vi "Controls on Tab.vi"(8 "error in (no error)":errorcluster, 11 "VI Refnum in":refnum<vi>) -> (0 "error out":errorcluster, 2 "ControlOnPages":refnum<vi>[][](array[refnum]), 3 "VI Refnum out":refnum<vi>)   [LabVIEW 2017, in "Toolbox.lvlib"]
uses:
  Toolbox.lvlib
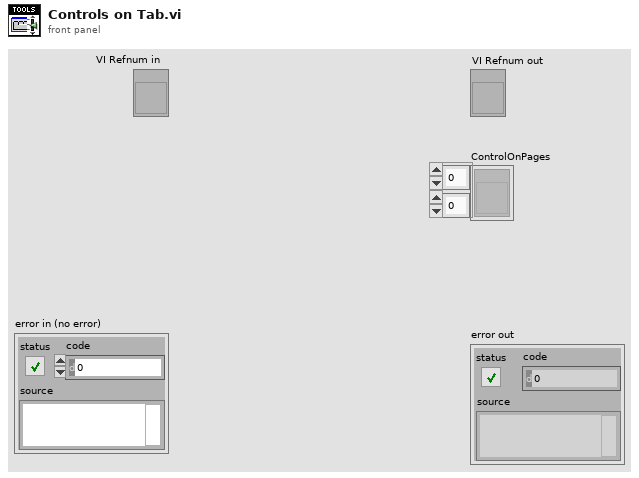
[diagram p1: front panel]
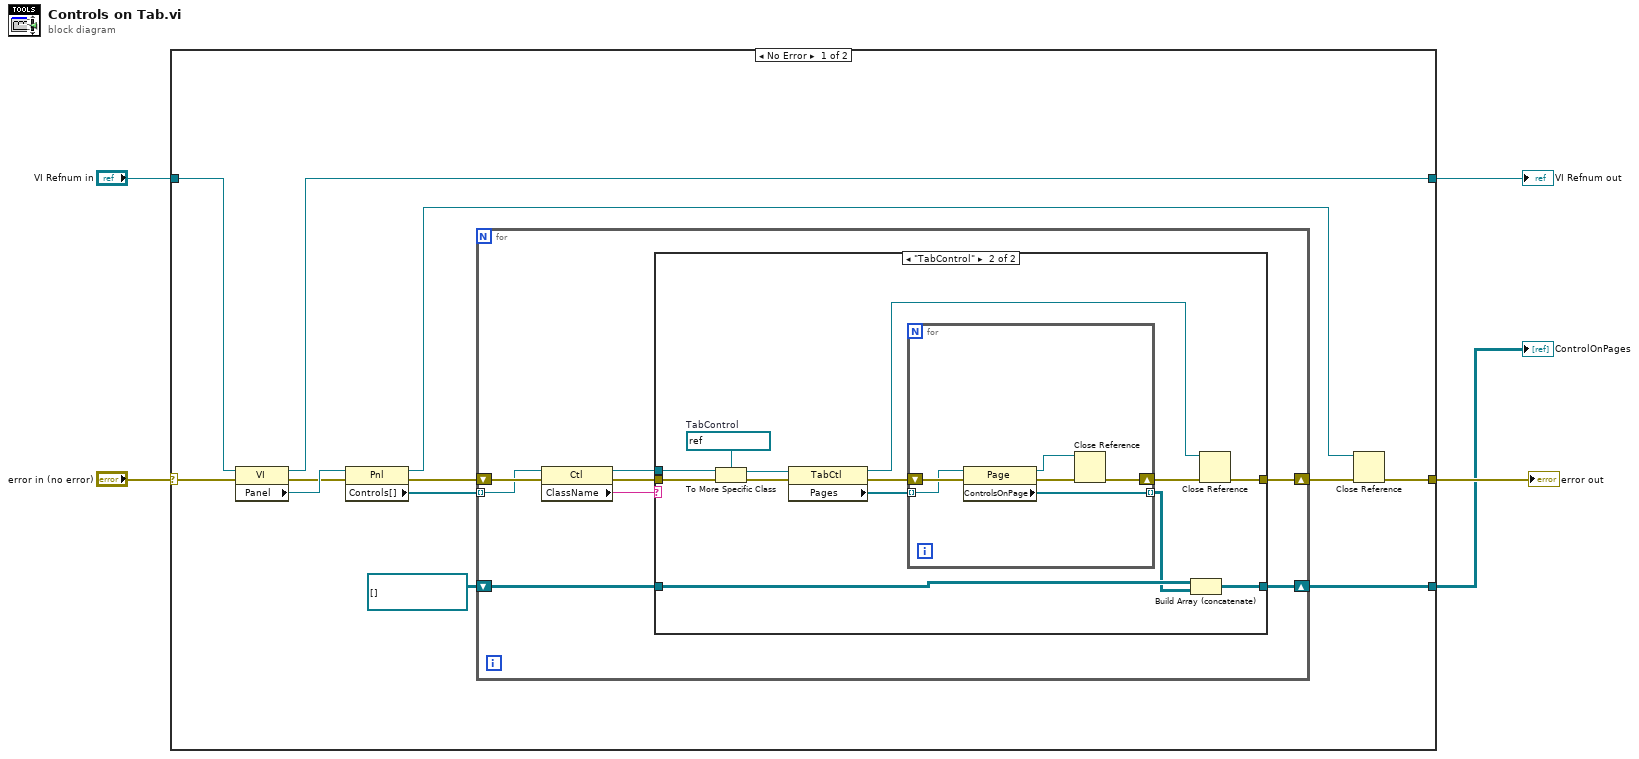
[diagram p0: block diagram]
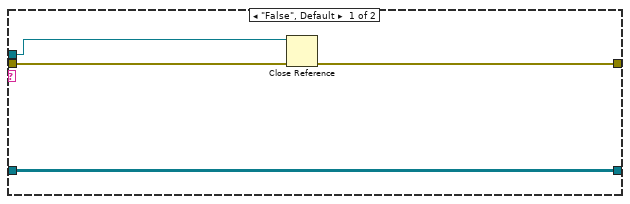
[diagram p2: hidden frame]
diagram:
  n1 = case shown="No Error" "error in (no error)" {
    selector: "error in (no error)" -> [w17 w50]
    tunnel: [w9 w50] -> w4
    tunnel: "VI Refnum in" -> [w16 w49]
    tunnel: [w12 w49] -> w2
    tunnel: [w7 _] -> w1
    frame No Error {
      n2 = property class="VI"(reference=w16, error in=w17) -> (reference out=w12:refnum<vi>, error out=w14:errorcluster, "Panel"=w15:refnum<vi>)
      n3 = property class="Pnl"(reference=w15, error in=w14) -> (reference out=w8:refnum<vi>, error out=w13:errorcluster, "Controls[]"=w10:refnum<vi>[])
      n4 = for {
        shift-right: [w22] -> w11
        shift-left: w13 -> [w25]
        tunnel: w10 -> [w23] mode=indexing
        shift-right: [w19] -> w7
        shift-left: refnum<vi>[][] [] -> [w18]
        n5 = property class="Ctl"(reference=w23, error in=w25) -> (reference out=w20:refnum<vi>, error out=w24:errorcluster, "ClassName"=w21:string)
        n6 = case shown="\"TabControl\"" w21 {
          tunnel: w24 -> [w29 w42]
          tunnel: [w28 w34] -> w22
          tunnel: w20 -> [w27 w38]
          tunnel: [w26 w32] -> w19
          tunnel: w18 -> [w26 w31]
          frame "False", Default {
            n7 = Close Reference(reference=w27, error in (no error)=w29) -> (error out=w28:errorcluster)
          }
          frame "TabControl" {
            w39 = refnum<vi> refnum  # TabControl
            n8 = To More Specific Class(target class=w39, reference=w38, error in=w42) -> (specific class reference=w37:refnum<vi>, error out=w40:errorcluster)
            n9 = property class="TabCtl"(reference=w37, error in=w40) -> (reference out=w33:refnum<vi>, error out=w41:errorcluster, "Pages"=w35:refnum<vi>[])
            n10 = for {
              shift-right: [w45] -> w36
              shift-left: w41 -> [w48]
              tunnel: w35 -> [w46] mode=indexing
              tunnel: [w43] -> w30 mode=indexing
              n11 = property class="Page"(reference=w46, error in=w48) -> (reference out=w44:refnum<vi>, error out=w47:errorcluster, "ControlsOnPage"=w43:refnum<vi>[])
              n12 = Close Reference(reference=w44, error in (no error)=w47) -> (error out=w45:errorcluster)
            }
            n13 = Build Array (concatenate)(w31, w30) -> (w32:refnum<vi>[][])
            n14 = Close Reference(reference=w33, error in (no error)=w36) -> (error out=w34:errorcluster)
          }
        }
      }
      n15 = Close Reference(reference=w8, error in (no error)=w11) -> (error out=w9:errorcluster)
    }
    frame Error {
    }
  }
  "error out" <- w4
  "VI Refnum out" <- w2
  "ControlOnPages" <- w1
